vi "Triangles set.vi"(0 "Triangle Info":T1) -> ()   [LabVIEW 2012]
panel:
  # "Operator Info"
  # "R"
  # "L"
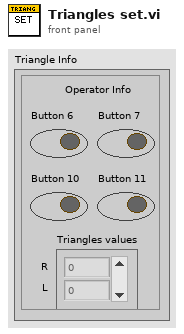
[diagram p1: front panel]
types:
  T1 = cluster{"Button 6":bool, "Button 7":bool, "Button 10":bool, "Button 11":bool, "Triangles values":dbl[]}
  T2 = typedef "WPI_MotorControlDeviceRef.ctl" = cluster{"DeviceStatus":errorcluster, "Type":enum16{"PWM", "CAN"}, "PWM":cluster{"Digital Module":T3, "PWM Channel":T4, "DeadBand":T5}, "CAN":cluster{"Device Number":u8, "Control Mode":T6, "Semaphore":T7, "Max Vout":dbl}, "Invert":bool, "TransformRef":T8, "InvTransformRef":T8}
  T3 = typedef "FPGA_TypedefDigitalModule.ctl" = enum16{"Digital Module 1", "Digital Module 2"}
  T4 = typedef "FPGA_DIOPWMChannel.ctl" = enum8{"PWM 1", "PWM 2", "PWM 3", "PWM 4", "PWM 5", "PWM 6", "PWM 7", "PWM 8", "PWM 9", "PWM 10", "Invalid"}
  T5 = typedef "WPI_PWMDeadband.ctl" = cluster{"Name":string, "maxPositivePwm":i32, "minPositivePwm":i32, "centerPwm":i32, "maxNegativePwm":i32, "minNegativePwm":i32, "angularRange":u16}
  T6 = typedef "WPI_CANJaguar_ControlMode.ctl" = enum8{"Percent VBus", "Current", "Speed", "Position", "Voltage"}
  T7 = typedef "Semaphore RefNum" = refnum<k1>
  T8 = typedef "WPI_PWMTransform_ConPane.ctl" = refnum<vi>
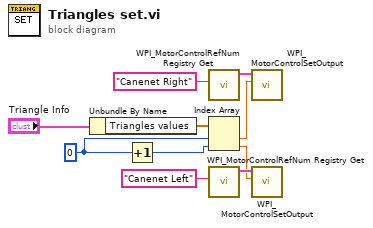
[diagram p0: block diagram]
diagram:
  w4 = 0
  n1 = Unbundle By Name("Triangle Info") -> ("Triangles values"=w3:dbl[])
  n2 = Increment(x=w4) -> (x+1=w5:i32)
  n3 = call <vilib>:"WPI_MotorControlRefNum Registry Get.vi"("refnum name"="Canenet Right") -> ("MotorControlDevRef"=w7:T2)  [unwired: 9 in, 1 out]
  n4 = Index Array(array=w3, index #1=w4, index #2=w5) -> (element #1=w2:dbl, element #2=w1:dbl)
  n5 = call <vilib>:"WPI_MotorControlRefNum Registry Get.vi"("refnum name"="Canenet Left") -> ("MotorControlDevRef"=w8:T2)  [unwired: 9 in, 1 out]
  n6 = call <vilib>:"WPI_MotorControlSetOutput.vi"("Output"=w2, "MotorControlDevRef"=w7) -> ()  [unwired: 7 in, 3 out]
  n7 = call <vilib>:"WPI_MotorControlSetOutput.vi"("Output"=w1, "MotorControlDevRef"=w8) -> ()  [unwired: 7 in, 3 out]
